vi "Geraetetype lesen.vi"(8 "error in (no error)":errorcluster caption="Fehler (Eingang, kein Fehler)", 11 "Steuerung PNS (Eingang)":refnum<class "Steuerung PNS.lvclass">) -> (0 "error out":errorcluster caption="Fehler (Ausgang)", 2 "Gerätetype":string, 3 "Steuerung PNS (Ausgang)":refnum<class "Steuerung PNS.lvclass">)   [LabVIEW 2020, in "Steuerung PNS.lvclass"]
uses:
  Steuerung PNS.lvclass
  Steuerung PNS.lvclass/Steuerung PNS.ctl
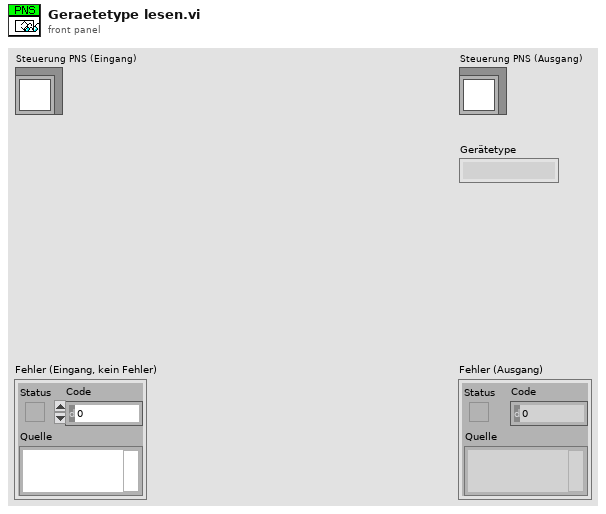
[diagram p1: front panel]
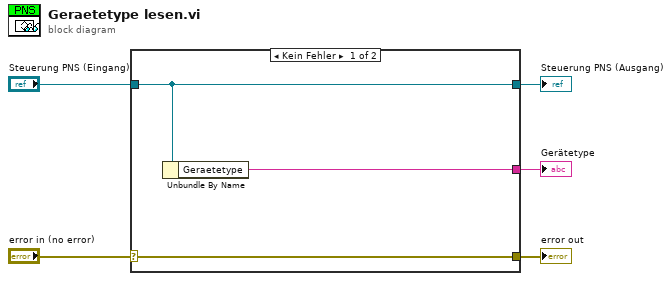
[diagram p0: block diagram]
diagram:
  n1 = case shown="Kein Fehler" "error in (no error)" {
    selector: "error in (no error)" -> [w8 w9]
    tunnel: [w8 w9] -> w4
    tunnel: [w7 w10] -> w2
    tunnel: "Steuerung PNS (Eingang)" -> [w7 w10]
    tunnel: [w6 _] -> w1
    frame No Error {
      n2 = Unbundle By Name(w7) -> ("Geraetetype"=w6:string)
    }
    frame Error {
    }
  }
  "error out" <- w4
  "Steuerung PNS (Ausgang)" <- w2
  "Gerätetype" <- w1
